vi "Test Monochromator.vi"   [LabVIEW 2024]
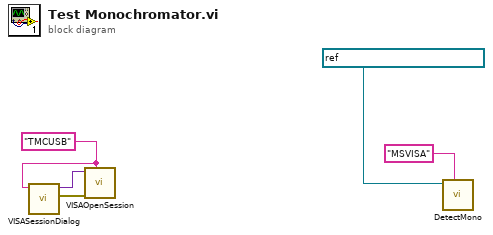
[diagram p0: block diagram]
diagram:
  w3 = "TMCUSB" ("Resource Type")
  n1 = call "VISASessionDialog.vi"("Resource Type"=w3) -> ("Error Out"=w5:errorcluster, "Variant"=w4:variant)  [unwired: 9 in]
  n2 = call "VISAOpenSession.vi"("Resource Type"=w3, "error in (no error)"=w5, "Variant"=w4) -> ()  [unwired: 7 in, 2 out]
  n3 = call "DetectMono.vi"("regular expression"="MSVISA", "Variant"=refnum<visa-resource-name> "SaraMONOCHROMATOR" ("VISA resource name")) -> ()  [unwired: 8 in, 2 out]
